vi "Initialize.vi"(8 "error in (no error)":errorcluster, 10 "Bitfile path":path, 11 "Device address":string) -> (0 "error out":errorcluster, 3 "FPGA Interface out":refnum<class "FPGA Interface.lvclass">)   [LabVIEW 2020, in "BCI-1553 API.lvlib" / "FPGA Interface.lvlib" / "FPGA Interface.lvclass"]
doc: "Opens a connection with a specific FPGA bitfile that has been compiled for communicating with the BCI-1553 modules."
uses:
  FPGA Interface.lvclass
  FPGA Interface.lvclass/FPGA Interface.ctl
  <vilib>/rvi/interface/common/niFpgaWaitOnOcc.vi
  <vilib>/Utility/error.llb/Error Cluster From Error Code.vi
  <vilib>/rvi/errors/niLvFpgaAdjustHostInterfaceError.vi
  <vilib>/rvi/interface/nirviMethod/nirviMethod.xnode
  <vilib>/FPGAPlugInAG/Dynamic/niLvFpga_ConfigureFifo_Dynamic.vi
  <vilib>/rvi/errors/niLvFpgaMergeErrorWithErrorCode.vi
  <vilib>/FPGAPlugInAG/Dynamic/niLvFpga_ReadFifo_Dynamic.vi
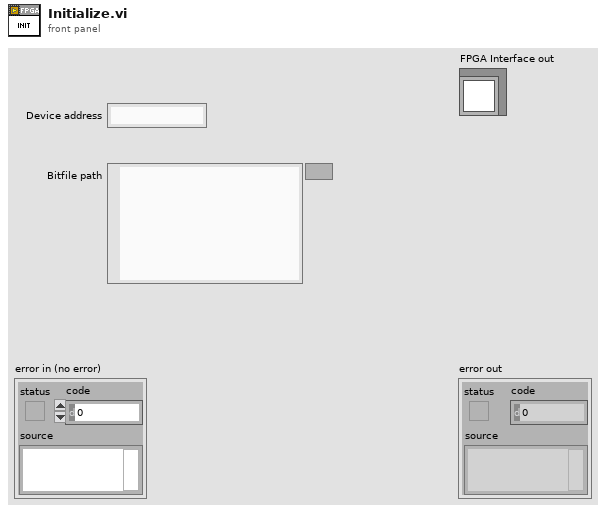
[diagram p1: front panel]
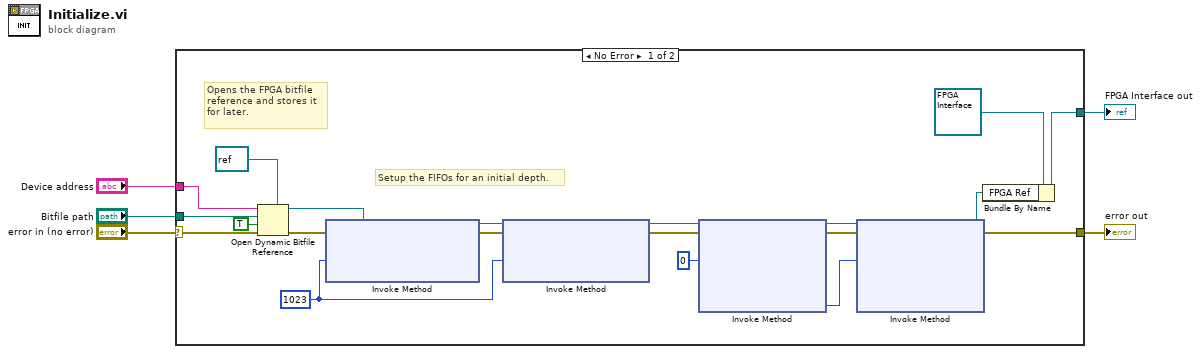
[diagram p0: block diagram]
diagram:
  n1 = case shown="No Error" "error in (no error)" {
    selector: "error in (no error)" -> [w25 w26]
    tunnel: [w8 w26] -> w4
    tunnel: [w19 _] -> w3
    tunnel: "Device address" -> [w24 _]
    tunnel: "Bitfile path" -> [w23 _]
    frame No Error {
      w14 = u32 1023 ("Requested Depth")
      # "Setup the FIFOs for an initial depth."
      # "Opens the FPGA bitfile\nreference and stores it\nfor later."
      n2 = Open Dynamic Bitfile Reference(0:w24, 1:w23, 2:TRUE ("Run When Loaded"), 3:w25, 4:refnum<k20> refnum ("Type")) -> (5:w17:refnum<k20>, 8:w15:errorcluster)
      n3 = xnode "Invoke Method"("FPGA VI Reference In"=w17, "error in"=w15, "Requested Depth"=w14) -> ("FPGA VI Reference Out"=w18:refnum<k20>, "error out"=w16:errorcluster)  [unwired: 1 out]
      n4 = xnode "Invoke Method"("FPGA VI Reference In"=w18, "error in"=w16, "Requested Depth"=w14) -> ("FPGA VI Reference Out"=w10:refnum<k20>, "error out"=w7:errorcluster)  [unwired: 1 out]
      n5 = xnode "Invoke Method"("FPGA VI Reference In"=w10, "error in"=w7, "Number of Elements"=u32 0) -> ("FPGA VI Reference Out"=w11:refnum<k20>, "error out"=w6:errorcluster, "Elements Remaining"=w12:u32)  [unwired: 1 in, 1 out]
      n6 = xnode "Invoke Method"("FPGA VI Reference In"=w11, "error in"=w6, "Number of Elements"=w12) -> ("FPGA VI Reference Out"=w9:refnum<k20>, "error out"=w8:errorcluster)  [unwired: 1 in, 2 out]
      n7 = Bundle By Name(cluster=refnum<class "FPGA Interface.lvclass"> refnum ("FPGA Interface in"), "FPGA Ref"=w9) -> (w19:refnum<class "FPGA Interface.lvclass">)
    }
    frame Error {
    }
  }
  "error out" <- w4
  "FPGA Interface out" <- w3
